vi "Build_Asylum_ScanForDevices.vi"() -> ()   [LabVIEW 2016]
panel:
  out "error out":errorcluster
  in  "error in (no error)":errorcluster
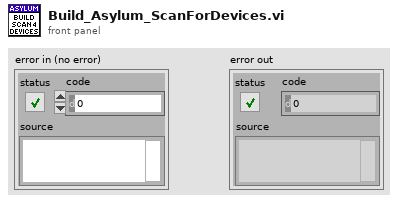
[diagram p1: front panel]
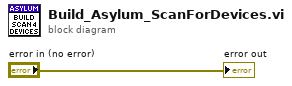
[diagram p0: block diagram]
diagram:
  "error out" <- "error in (no error)"
